vi "Xsens DeltaQ (SubVI).vi"(1 "DATA in (Hex)":string) -> (0 "DeltaQ":T1 {"DQ2" format="%#.7f"})   [LabVIEW 2019]
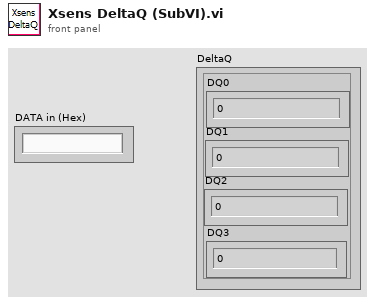
[diagram p1: front panel]
types:
  T1 = cluster{"DQ0":dbl, "DQ1":dbl, "DQ2":dbl, "DQ3":dbl}
  T2 = cluster{"DBL":dbl, "DBL":dbl, "DBL":dbl, "DBL":dbl}
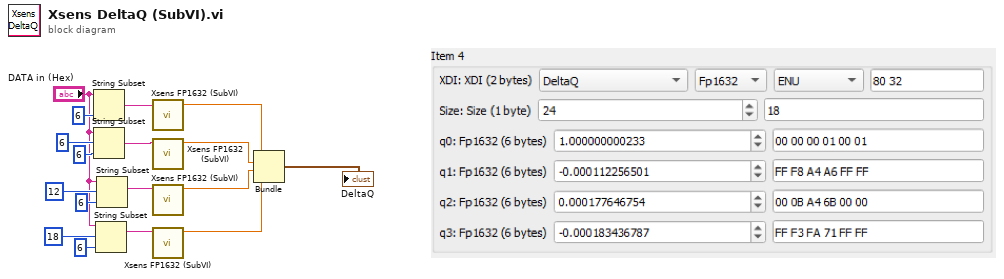
[diagram p0: block diagram]
diagram:
  n1 = String Subset(string="DATA in (Hex)", length (rest)=6 ("length (rest)")) -> (substring=w1:string)  [unwired: 1 in]
  n2 = String Subset(string="DATA in (Hex)", offset (0)=6, length (rest)=6 ("length (rest)")) -> (substring=w9:string)
  n3 = String Subset(string="DATA in (Hex)", offset (0)=18, length (rest)=6 ("length (rest)")) -> (substring=w6:string)
  n4 = String Subset(string="DATA in (Hex)", offset (0)=12, length (rest)=6 ("length (rest)")) -> (substring=w7:string)
  n5 = call "Xsens FP1632 (SubVI).vi"("6 Byte Hex String"=w1) -> ("DBL"=w2:dbl)  [unwired: 10 in]
  n6 = call "Xsens FP1632 (SubVI).vi"("6 Byte Hex String"=w9) -> ("DBL"=w8:dbl)  [unwired: 10 in]
  n7 = call "Xsens FP1632 (SubVI).vi"("6 Byte Hex String"=w7) -> ("DBL"=w5:dbl)  [unwired: 10 in]
  n8 = call "Xsens FP1632 (SubVI).vi"("6 Byte Hex String"=w6) -> ("DBL"=w4:dbl)  [unwired: 10 in]
  n9 = Bundle("DBL"=w2, "DBL"=w8, "DBL"=w5, "DBL"=w4) -> (→"DeltaQ":T2)  [unwired: 1 in]
